vi "Set Data Word Format.vi"(8 "error in":errorcluster, 10 "data word format":T1="Decimal", 11 "logging section":T2=18446744073709551615 format="%.0x") -> (0 "error out":errorcluster, 3 "logging section out":T2 format="%.0x")   [LabVIEW 2020, in "AIM MIL-STD-1553 Scripting.lvlib"]
doc: "Specifies the format of data words in the log file."
uses:
  AIM MIL-STD-1553 Scripting.lvlib
  <vilib>/NI VeriStand/Custom Device API/Custom Device Item Ref.ctl
  Shared/Data Word Format.ctl
  Constants.vi
  <vilib>/NI VeriStand/Custom Device API/Set Item Property (String).vi
  <vilib>/NI VeriStand/Custom Device API/Custom Device API.lvlib
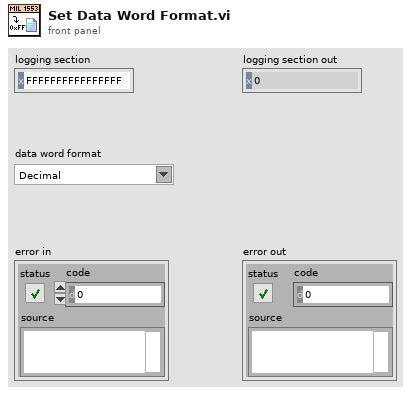
[diagram p1: front panel]
types:
  T1 = typedef "Data Word Format.ctl" = string
  T2 = typedef "Custom Device API.lvlib/Custom Device Item Ref.ctl" = u64
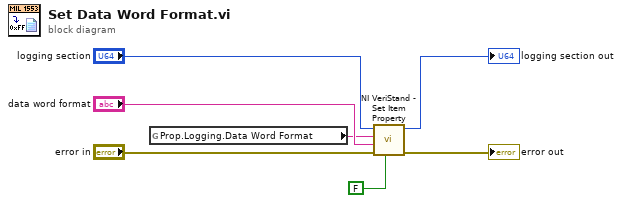
[diagram p0: block diagram]
diagram:
  n1 = global read "Constants.vi" "Prop.Logging.Data Word Format"() -> (w1:string)
  n2 = call-poly <vilib>:"NI VeriStand - Set Item Property.vi"("Binary String (T)"=FALSE, "error in (no error)"="error in", "Value"="data word format", "Property Name"=w1, "Item Ref in"="logging section") -> ("error out"=→"error out":errorcluster, "Item Ref out"=→"logging section out":T2)  [unwired: 4 in, 1 out]
